vi "Adapt triangles.vi"(1 "Triangles in (indexed type)":T2[](array[typedef])) -> (0 "Triangles out (full type)":T1[](array[typedef]))   [LabVIEW 2014]
doc: "This VI must be run after any alteration to the triangles geometry involving scaling and rotation.\nThere is no need to run this VI after applying a translation."
uses:
  Typedefs/Triangle, indexed.ctl
  Typedefs/Triangle.ctl
panel:
  # "PN 29/03/2015"
  # "Vertices"
  # "Edges"
  # "Unit normal"
  # "Edge unit normals"
  # "Vertices"
  # "Indices"
  # "Unit normal"
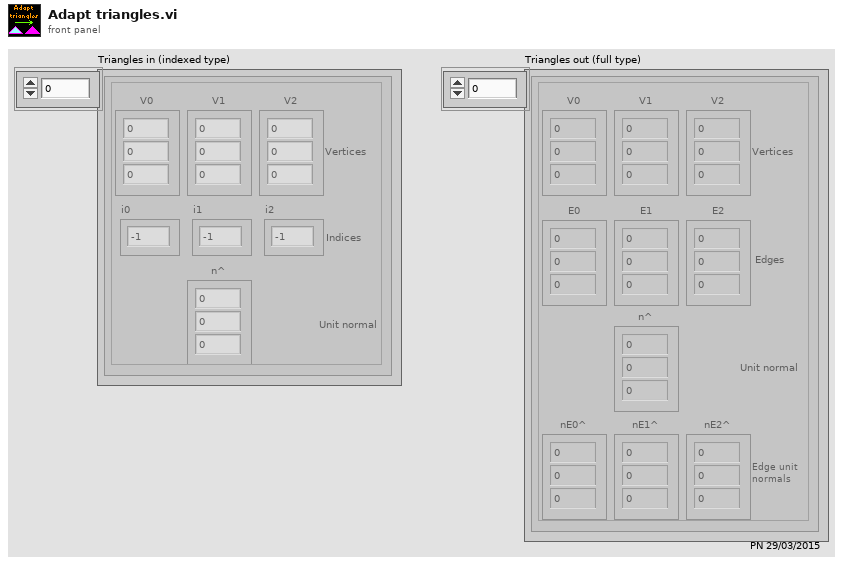
[diagram p1: front panel]
types:
  T1 = typedef "Triangle.ctl" = cluster{"V0":sgl[], "V1":sgl[], "V2":sgl[], "E0":sgl[], "E1":sgl[], "E2":sgl[], "n^":sgl[], "nE0^":sgl[], "nE1^":sgl[], "nE2^":sgl[]}
  T2 = typedef "Triangle, indexed.ctl" = cluster{"V0":sgl[], "V1":sgl[], "V2":sgl[], "n^":sgl[], "i0":i32, "i1":i32, "i2":i32}
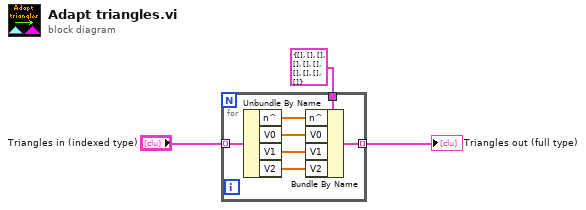
[diagram p0: block diagram]
diagram:
  n1 = for {
    tunnel: T1 {"V0"=[], "V1"=[], "V2"=[], "E0"=[], "E1"=[], "E2"=[], "n^"=[], "nE0^"=[], "nE1^"=[], "nE2^"=[]} ("Triangle out") -> [w10]
    tunnel: "Triangles in (indexed type)" -> [w5] mode=indexing
    tunnel: [w4] -> w1 mode=indexing
    n2 = Unbundle By Name(w5) -> ("n^"=w9:sgl[], "V0"=w8:sgl[], "V1"=w7:sgl[], "V2"=w6:sgl[])
    n3 = Bundle By Name(cluster=w10, "n^"=w9, "V0"=w8, "V1"=w7, "V2"=w6) -> (w4:T1)
  }
  "Triangles out (full type)" <- w1
